vi "dialOutput.vi"() -> ()   [LabVIEW 2013]
panel:
  out "Numeric 2":dbl
  in  "stop":bool
  out "Numeric":dbl
  in  "Dial":dbl(knob) scale=0.0..10.0
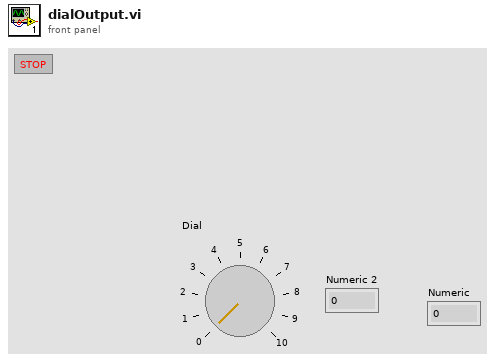
[diagram p1: front panel]
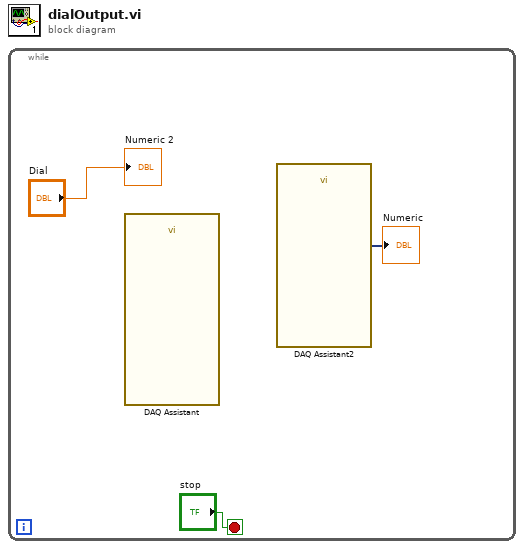
[diagram p0: block diagram]
diagram:
  n1 = while {
    stop <- "stop" stop-if-true
    n2 = call "DAQ Assistant"() -> ()  [unwired: 18 in, 2 out]
    n3 = call "DAQ Assistant2"() -> ("data"=→"Numeric":dynamicdata)  [unwired: 17 in, 2 out]
    "Numeric 2" <- "Dial"
  }
